vi "TS Result Decoding.vi"(11 "StepResult":refnum<k7>) -> (2 "Test Number":string, 3 "Test Result":string)   [LabVIEW 2023]
panel:
  out "error out":errorcluster
  in  "error in (no error)":errorcluster
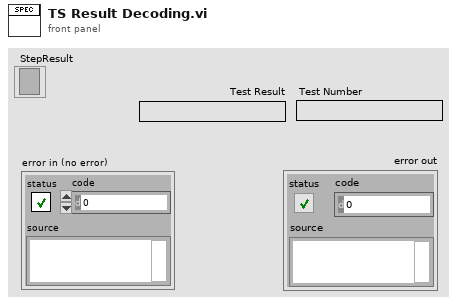
[diagram p1: front panel]
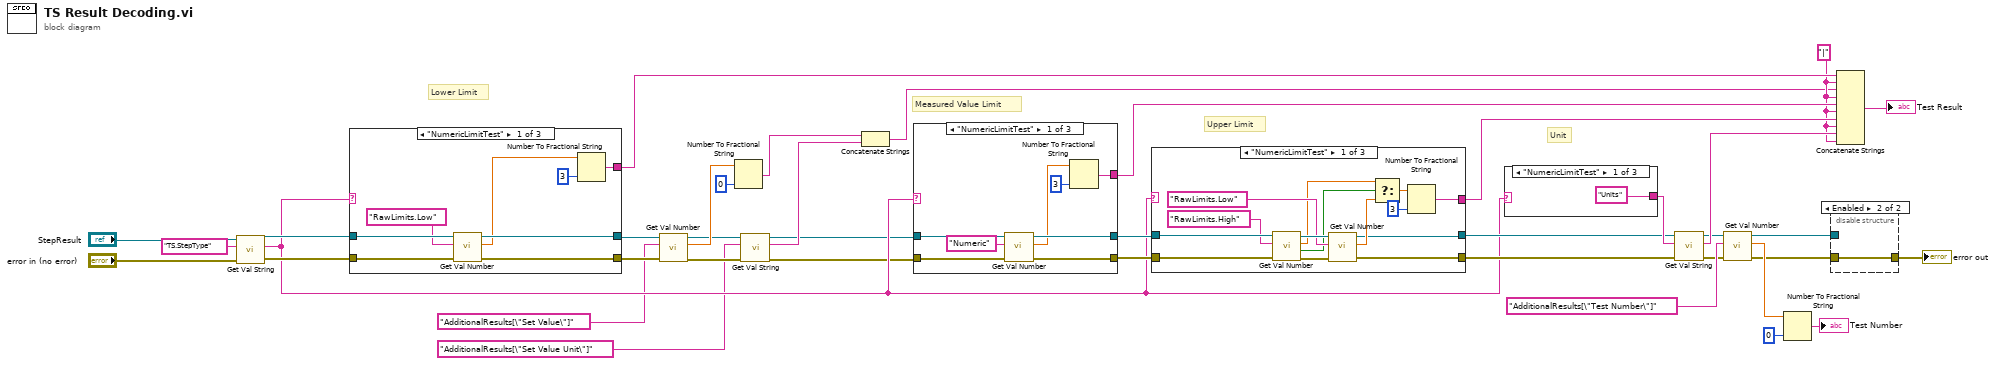
[diagram p0: block diagram]
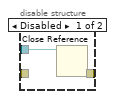
[diagram p2: hidden frame]
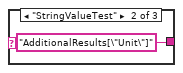
[diagram p3: hidden frame]
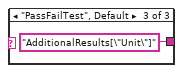
[diagram p4: hidden frame]
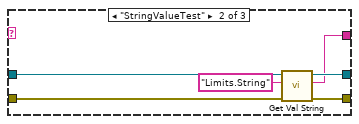
[diagram p5: hidden frame]
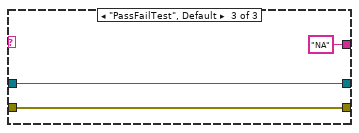
[diagram p6: hidden frame]
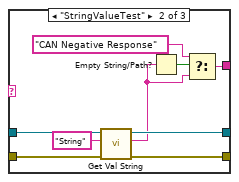
[diagram p7: hidden frame]
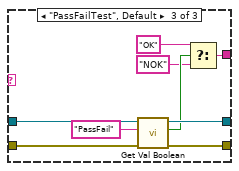
[diagram p8: hidden frame]
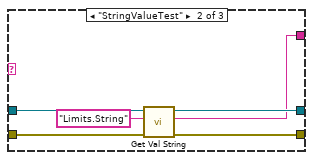
[diagram p9: hidden frame]
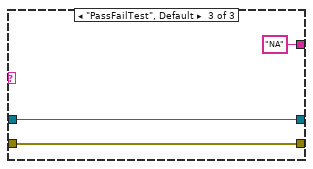
[diagram p10: hidden frame]
diagram:
  w14 = "|" ("string")
  # "Unit"
  # "Upper Limit"
  # "Measured Value Limit"
  # "Lower Limit"
  n1 = call "Get Val String.vi"("error in (no error)"="error in (no error)", "Lookup String"="TS.StepType", "Property Object In"="StepResult") -> ("error out"=w37:errorcluster, "String"=w29:string, "Property Object Out"=w38:refnum<k7>)  [unwired: 5 in, 1 out]
  n2 = case shown="\"NumericLimitTest\"" w29 {
    tunnel: [w47 w52 w56] -> w11
    tunnel: [w46 w49 w55] -> w12
    tunnel: w37 -> [w45 w50 w55]
    tunnel: w38 -> [w44 w51 w56]
    tunnel: [w43 w48 "NA"] -> w34
    frame "NumericLimitTest" {
      n3 = call "Get Val Number.vi"("error in (no error)"=w45, "Lookup String"="RawLimits.Low", "Property Object In"=w44) -> ("error out"=w46:errorcluster, "Number"=w40:dbl, "Property Object Out"=w47:refnum<k7>)  [unwired: 6 out]
      n4 = Number To Fractional String(number=w40, precision (6)=i16 3) -> (F-format string=w43:string)  [unwired: 2 in]
    }
    frame "StringValueTest" {
      n5 = call "Get Val String.vi"("error in (no error)"=w50, "Lookup String"="Limits.String", "Property Object In"=w51) -> ("error out"=w49:errorcluster, "String"=w48:string, "Property Object Out"=w52:refnum<k7>)  [unwired: 5 in, 1 out]
    }
    frame "PassFailTest", Default {
    }
  }
  n6 = call "Get Val Number.vi"("error in (no error)"=w12, "Lookup String"="AdditionalResults[\"Set Value\"]", "Property Object In"=w11) -> ("error out"=w6:errorcluster, "Number"=w9:dbl, "Property Object Out"=w3:refnum<k7>)  [unwired: 5 in, 1 out]
  n7 = Number To Fractional String(number=w9, precision (6)=i16 0) -> (F-format string=w13:string)  [unwired: 2 in]
  n8 = call "Get Val String.vi"("error in (no error)"=w6, "Lookup String"="AdditionalResults[\"Set Value Unit\"]", "Property Object In"=w3) -> ("error out"=w5:errorcluster, "String"=w7:string, "Property Object Out"=w2:refnum<k7>)  [unwired: 5 in, 1 out]
  n9 = Concatenate Strings(w13, w7) -> (w1:string)
  n10 = case shown="\"NumericLimitTest\"" w29 {
    tunnel: [w64 w70 w80] -> w36
    tunnel: [w63 w69 w79] -> w35
    tunnel: w5 -> [w62 w72 w81]
    tunnel: w2 -> [w61 w73 w82]
    tunnel: [w60 w65 w74] -> w15
    frame "NumericLimitTest" {
      n11 = call "Get Val Number.vi"("error in (no error)"=w62, "Lookup String"="Numeric", "Property Object In"=w61) -> ("error out"=w63:errorcluster, "Number"=w57:dbl, "Property Object Out"=w64:refnum<k7>)  [unwired: 6 out]
      n12 = Number To Fractional String(number=w57, precision (6)=i16 3) -> (F-format string=w60:string)  [unwired: 2 in]
    }
    frame "StringValueTest" {
      n13 = call "Get Val String.vi"("error in (no error)"=w72, "Lookup String"="String", "Property Object In"=w73) -> ("error out"=w69:errorcluster, "String"=w66:string, "Property Object Out"=w70:refnum<k7>)  [unwired: 5 in, 1 out]
      n14 = Empty String/Path?(string/path=w66) -> (empty?=w68:bool)
      n15 = Select(t="CAN Negative Response", s=w68, f=w66) -> (s? t:f=w65:string)
    }
    frame "PassFailTest", Default {
      n16 = call "Get Val Boolean.vi"("error in (no error)"=w81, "Lookup String"="PassFail", "Property Object In"=w82) -> ("error out"=w79:errorcluster, "Boolean"=w77:bool, "Property Object Out"=w80:refnum<k7>)  [unwired: 5 in, 1 out]
      n17 = Select(t="OK", s=w77, f="NOK") -> (s? t:f=w74:string)
    }
  }
  n18 = case shown="\"NumericLimitTest\"" w29 {
    tunnel: [w84 w100 w105] -> w31
    tunnel: [w83 w99 w104] -> w30
    tunnel: w35 -> [w96 w101 w104]
    tunnel: w36 -> [w93 w102 w105]
    tunnel: [w95 w97 "NA"] -> w19
    frame "NumericLimitTest" {
      n19 = call "Get Val Number.vi"("error in (no error)"=w96, "Lookup String"="RawLimits.High", "Property Object In"=w93) -> ("error out"=w90:errorcluster, "Exists"=w88:bool, "Number"=w87:dbl, "Property Object Out"=w91:refnum<k7>)  [unwired: 5 out]
      n20 = call "Get Val Number.vi"("error in (no error)"=w90, "Lookup String"="RawLimits.Low", "Property Object In"=w91) -> ("error out"=w83:errorcluster, "Number"=w86:dbl, "Property Object Out"=w84:refnum<k7>)  [unwired: 6 out]
      n21 = Select(t=w87, s=w88, f=w86) -> (s? t:f=w85:dbl)
      n22 = Number To Fractional String(number=w85, precision (6)=i16 3) -> (F-format string=w95:string)  [unwired: 2 in]
    }
    frame "StringValueTest" {
      n23 = call "Get Val String.vi"("error in (no error)"=w101, "Lookup String"="Limits.String", "Property Object In"=w102) -> ("error out"=w99:errorcluster, "String"=w97:string, "Property Object Out"=w100:refnum<k7>)  [unwired: 5 in, 1 out]
    }
    frame "PassFailTest", Default {
    }
  }
  n24 = case shown="\"NumericLimitTest\"" w29 {
    tunnel: ["Units" ("Lookup String") "AdditionalResults[\"Unit\"]" ("Lookup String") "AdditionalResults[\"Unit\"]" ("Lookup String")] -> w32
    frame "NumericLimitTest" {
    }
    frame "StringValueTest" {
    }
    frame "PassFailTest", Default {
    }
  }
  n25 = call "Get Val String.vi"("error in (no error)"=w30, "Lookup String"=w32, "Property Object In"=w31) -> ("error out"=w23:errorcluster, "String"=w28:string, "Property Object Out"=w25:refnum<k7>)  [unwired: 5 in, 1 out]
  n26 = call "Get Val Number.vi"("error in (no error)"=w23, "Lookup String"="AdditionalResults[\"Test Number\"]", "Property Object In"=w25) -> ("error out"=w8:errorcluster, "Number"=w22:dbl, "Property Object Out"=w24:refnum<k7>)  [unwired: 5 in, 1 out]
  n27 = Number To Fractional String(number=w22, precision (6)=i16 0) -> (F-format string=→"Test Number":string)  [unwired: 2 in]
  n28 = disable-structure shown="Enabled" {
    disable-tunnel: w24 -> [w110 _]
    disable-tunnel: [w109 w111] -> w27
    disable-tunnel: w8 -> [_ w111]
    frame Disabled {
      n29 = Close Reference(reference=w110) -> (error out=w109:errorcluster)  [unwired: 1 in]
    }
    frame Enabled {
    }
  }
  "error out" <- w27
  n30 = Concatenate Strings(w34, w14, w1, w14, w15, w14, w19, w14, w28, w14) -> (→"Test Result":string)
